vi "samletrev1.vi"() -> ()   [LabVIEW 2019]
uses:
  <vilib>/myRIO/Instrument Drivers/Onboard IO/AI/typedefs/AI Reference.ctl
  <vilib>/myRIO/Common/Instrument Driver Framework/Utilities/typedefs/myRIO Generic Hardware Reference.ctl
  <vilib>/myRIO/Common/Instrument Driver Framework/Utilities/typedefs/Hardware Version Enum.ctl
  <vilib>/myRIO/Common/Instrument Driver Framework/Utilities/typedefs/myRIO v1.0 Reference.ctl
  <vilib>/myRIO/Common/Instrument Driver Framework/Utilities/typedefs/Generic FPGA Reference.ctl
  <vilib>/myRIO/Common/Instrument Driver Framework/myRIO v1.0/AI/typedefs/AI Channels List.ctl
  <vilib>/myRIO/Common/Instrument Driver Framework/myRIO v1.0/AI/typedefs/AI Channels Enum.ctl
  <vilib>/myRIO/Common/Instrument Driver Framework/Utilities/typedefs/Analog Scaling Constants List.ctl
  <vilib>/myRIO/Common/Instrument Driver Framework/Utilities/typedefs/Analog Scaling Constants.ctl
  <vilib>/userdefined/High Color/nirio_resource_hc.ctl
  <vilib>/myRIO/Common/Instrument Driver Framework/myRIO v1.0/Encoder/typedefs/Encoder Signal Mode.ctl
  <vilib>/myRIO/Instrument Drivers/Onboard IO/Encoder/typedefs/Encoder Reference.ctl
  <vilib>/myRIO/Common/Instrument Driver Framework/myRIO v1.0/Encoder/typedefs/Encoder Channels Enum.ctl
  <vilib>/myRIO/Common/Instrument Driver Framework/myRIO v1.0/Encoder/typedefs/Encoder Configuration v1.0.ctl
  <vilib>/myRIO/Instrument Drivers/Onboard IO/PWM/typedefs/PWM Reference.ctl
  <vilib>/myRIO/Common/Instrument Driver Framework/myRIO v1.0/PWM/typedefs/PWM Channels Enum.ctl
  <vilib>/myRIO/Instrument Drivers/Onboard IO/PWM/typedefs/PWM Configuration.ctl
  <vilib>/myRIO/Common/Instrument Driver Framework/Utilities/vis/Is FPGA Ref Available.vi
  <vilib>/myRIO/Common/Instrument Driver Framework/myRIO v1.0/AI/vis/myRIO v1.1 Open AI.vi
  <vilib>/myRIO/Instrument Drivers/Onboard IO/AI/vis/Read.vi
  <vilib>/myRIO/Common/Instrument Driver Framework/myRIO v1.0/Encoder/vis/myRIO v1.1 Open Encoder.vi
  <vilib>/myRIO/Instrument Drivers/Onboard IO/Encoder/vis/Read.vi
  <vilib>/myRIO/Common/Instrument Driver Framework/myRIO v1.0/PWM/vis/myRIO v1.1 Open PWM.vi
  <vilib>/myRIO/Common/Instrument Driver Framework/Utilities/vis/Validate Channels.vi
  <vilib>/myRIO/Common/Instrument Driver Framework/myRIO v1.0/AI/vis/myRIO v1.0 Reserve AI.vi
  <vilib>/myRIO/Common/Instrument Driver Framework/myRIO v1.0/Encoder/vis/myRIO v1.0 Reserve Encoder.vi
  <vilib>/myRIO/Common/Instrument Driver Framework/myRIO v1.0/PWM/vis/myRIO v1.0 Reserve PWM.vi
  <vilib>/myRIO/Common/Instrument Driver Framework/myRIO v1.0/PWM/vis/myRIO v1.0 Close PWM.vi
  <vilib>/myRIO/Common/Instrument Driver Framework/myRIO v1.0/AI/vis/myRIO v1.0 Build MUX Configuration AI.vi
  <vilib>/myRIO/Common/Instrument Driver Framework/myRIO v1.0/Resource Manager/vis/myRIO v1.0 Reserve Channel List.vi
  <vilib>/myRIO/Common/Instrument Driver Framework/myRIO v1.0/Encoder/vis/myRIO v1.0 Build MUX Configuration Encoder.vi
  <vilib>/myRIO/Common/Instrument Driver Framework/myRIO v1.0/PWM/vis/myRIO v1.0 Build MUX Configuration PWM.vi
  <vilib>/myRIO/Common/Instrument Driver Framework/myRIO v1.0/PWM/vis/myRIO v1.0 Unreserve PWM.vi
  <vilib>/myRIO/Common/Instrument Driver Framework/myRIO v1.0/Resource Manager/vis/myRIO v1.0 Reserve Channel.vi
  <vilib>/myRIO/Common/Instrument Driver Framework/myRIO v1.0/Resource Manager/vis/myRIO v1.0 Unreserve Channel.vi
  <vilib>/myRIO/Common/Instrument Driver Framework/myRIO v1.0/Resource Manager/vis/myRIO v1.0 Create Configuration List.vi
  <vilib>/myRIO/Common/Instrument Driver Framework/myRIO v1.0/Resource Manager/vis/myRIO v1.0 Unreserve Channel List.vi
  <vilib>/myRIO/Common/Instrument Driver Framework/myRIO v1.0/Resource Manager/vis/myRIO v1.0 Build Mutex Name.vi
  <vilib>/Utility/VariantDataType/GetNumericInfo.vi
  <vilib>/Utility/error.llb/Error Cluster From Error Code.vi
  <vilib>/myRIO/Common/Instrument Driver Framework/myRIO v1.0/myRIO v1.1 Open.vi
  <vilib>/myRIO/Common/Instrument Driver Framework/Utilities/vis/IO Manager.vi
  <vilib>/myRIO/Common/Instrument Driver Framework/Utilities/vis/Configuration Manager.vi
  <vilib>/myRIO/Common/Instrument Driver Framework/myRIO v1.0/Resource Manager/vis/myRIO v1.0 Configure IO.vi
  <vilib>/myRIO/Common/Instrument Driver Framework/myRIO v1.0/myRIO v1.0 Close.vi
  <vilib>/myRIO/Common/Instrument Driver Framework/myRIO v1.0/PWM/vis/myRIO v1.0 Write PWM.vi
  <vilib>/myRIO/Common/Instrument Driver Framework/myRIO v1.0/PWM/vis/myRIO v1.0 Shutdown PWM.vi
  <vilib>/myRIO/Common/Instrument Driver Framework/myRIO v1.0/Encoder/vis/myRIO v1.0 Configure Encoder.vi
  <vilib>/myRIO/Common/Instrument Driver Framework/myRIO v1.0/Encoder/vis/myRIO v1.0 Read Encoder.vi
  <vilib>/myRIO/Common/Instrument Driver Framework/myRIO v1.0/AI/vis/myRIO v1.0 Get Scaling Constants AI.vi
  <vilib>/myRIO/Common/Instrument Driver Framework/myRIO v1.0/AI/vis/myRIO v1.0 Read AI.vi
  <vilib>/addons/control/pid/pid.llb/PID (DBL).vi
  <vilib>/myRIO/Instrument Drivers/Onboard IO/PWM/vis/myRIO PWM Open.xnode
  <vilib>/myRIO/Express VI/Onboard IO/Encoder/Encoder Express VI.xnode
  <vilib>/myRIO/Instrument Drivers/Onboard IO/Encoder/vis/myRIO Encoder Open.xnode
  <vilib>/myRIO/Common/Instrument Driver Framework/myRIO v1.0/Encoder/typedefs/Encoder Count Direction Enum.ctl
  <vilib>/myRIO/Express VI/Onboard IO/AI/AI Express VI.xnode
  <vilib>/myRIO/Instrument Drivers/Onboard IO/AI/vis/myRIO AI Open.xnode
  <vilib>/myRIO/Instrument Drivers/Onboard IO/PWM/PWM.lvlib
  <vilib>/myRIO/Instrument Drivers/Onboard IO/Encoder/Encoder.lvlib
  <vilib>/ptbypt/NI_PtbyPt.lvlib
  <vilib>/myRIO/Instrument Drivers/Onboard IO/AI/AI.lvlib
  <vilib>/addons/control/pid/NI_PID_pid.lvlib
panel:
  in  "y":dbl
  out "output":dbl format="%.2f"
  in  "PWM-treshold":dbl format="%#_13g"
  out "PWM-sig":dbl format="%.2f"
  in  "1-output range":cluster{"output high":dbl, "output low":dbl}={"output high"=100.0, "output low"=-100.0} {"output low" format="%.2f"; "output high" format="%.2f"}
  in  "PID-1 gains":T1={"proportional gain (Kc)"=1.0, "integral time (Ti, min)"=0.01, "derivative time (Td, min)"=0.0} {"derivative time (Td, min)" format="%.3f"; "integral time (Ti, min)" format="%.3f"; "proportional gain (Kc)" format="%.3f"}
  out "x(F.R) test":dbl
  out "x(F.L) test":dbl
  in  "stop":bool
  out "Front  Left(F.L)":T2(graph)
  out "Sensor 1":dbl=0.0038137989155123176 format="%0.5f"
  in  "ZERO ALL SENSORS":bool
  in  "STOP SYSTEM":bool
  out "Sensor 2":dbl=0.0038137989155123176 format="%0.5f"
  out "Front  Right(F.L)":T2(graph)
  out "Sensor 3":dbl=0.0038137989155123176 format="%0.5f"
  out "Back Left(F.L)":T2(graph)
  out "Sensor 4":dbl=0.0038137989155123176 format="%0.5f"
  out "Back Right(F.L)":T2(graph)
  out "Sensor 5":dbl=0.0038137989155123176 format="%0.5f"
  out "Front Left(F.R)":T2(graph)
  out "Sensor 6":dbl=0.0038137989155123176 format="%0.5f"
  out "Front Right(F.R)":T2(graph)
  out "Sensor 7":dbl=0.0038137989155123176 format="%0.5f"
  out "Back Left(F.R)":T2(graph)
  out "Sensor 8":dbl=0.0038137989155123176 format="%0.5f"
  out "Back Right(F.R)":T2(graph)
  out "Sensor 9":dbl=0.0038137989155123176 format="%0.5f"
  out "Axial(L)":T2(graph)
  out "Sensor 10":dbl=0.0038137989155123176 format="%0.5f"
  out "Axial(R)":T2(graph)
  in  "Cal(F.L)":dbl[](array[numeric])
  out "Kg(L)":dbl[](array[numeric])
  out "Sum(L)":dbl
  in  "Cal(F.R)":dbl[](array[numeric])
  out "Kg (R)":dbl[](array[numeric])
  out "Sum(R)":dbl
  out "x(F.R)":dbl
  out "y(F.R)":dbl
  out "sum(F.R)":dbl
  out "Sum (F.L)":dbl
  out "y(F.L)":dbl
  out "x(F.L)":dbl
  out "Cop Left":cluster{dbl[], dbl[]}(graph)
  out "Cop Right":cluster{dbl[], dbl[]}(graph)
  in  "x Right":dbl[](array[numeric])
  in  "kal Right":dbl=1.0
  in  "x Left":dbl[](array[numeric])
  in  "kal left":dbl=1.0
  in  "Stop":bool
  in  "Reset Counter":bool
  out "Counter Value Right":i32
  out "Pulstime Right":u32
  out "km/h Right belt":dbl(knob) scale=0.0..15.0
  out "km/h 2":dbl format="%#_2g"
  out "Counter Value left":i32
  out "Pulstime left":u32
  out "km/h left belt":dbl(knob) scale=0.0..15.0
  out "km/h":dbl format="%#_2g"
  in  "STOP RIGHT MOTOR":bool
  in  "RIGHT MOTOR DUTY CYCLE":dbl(slide)=50.00000000000001 scale=0.0..100.0
  in  "STOP LEFT MOTOR":bool
  in  "LEFT MOTOR DUTY CYCLE":dbl(slide)=50.00000000000001 scale=0.0..100.0
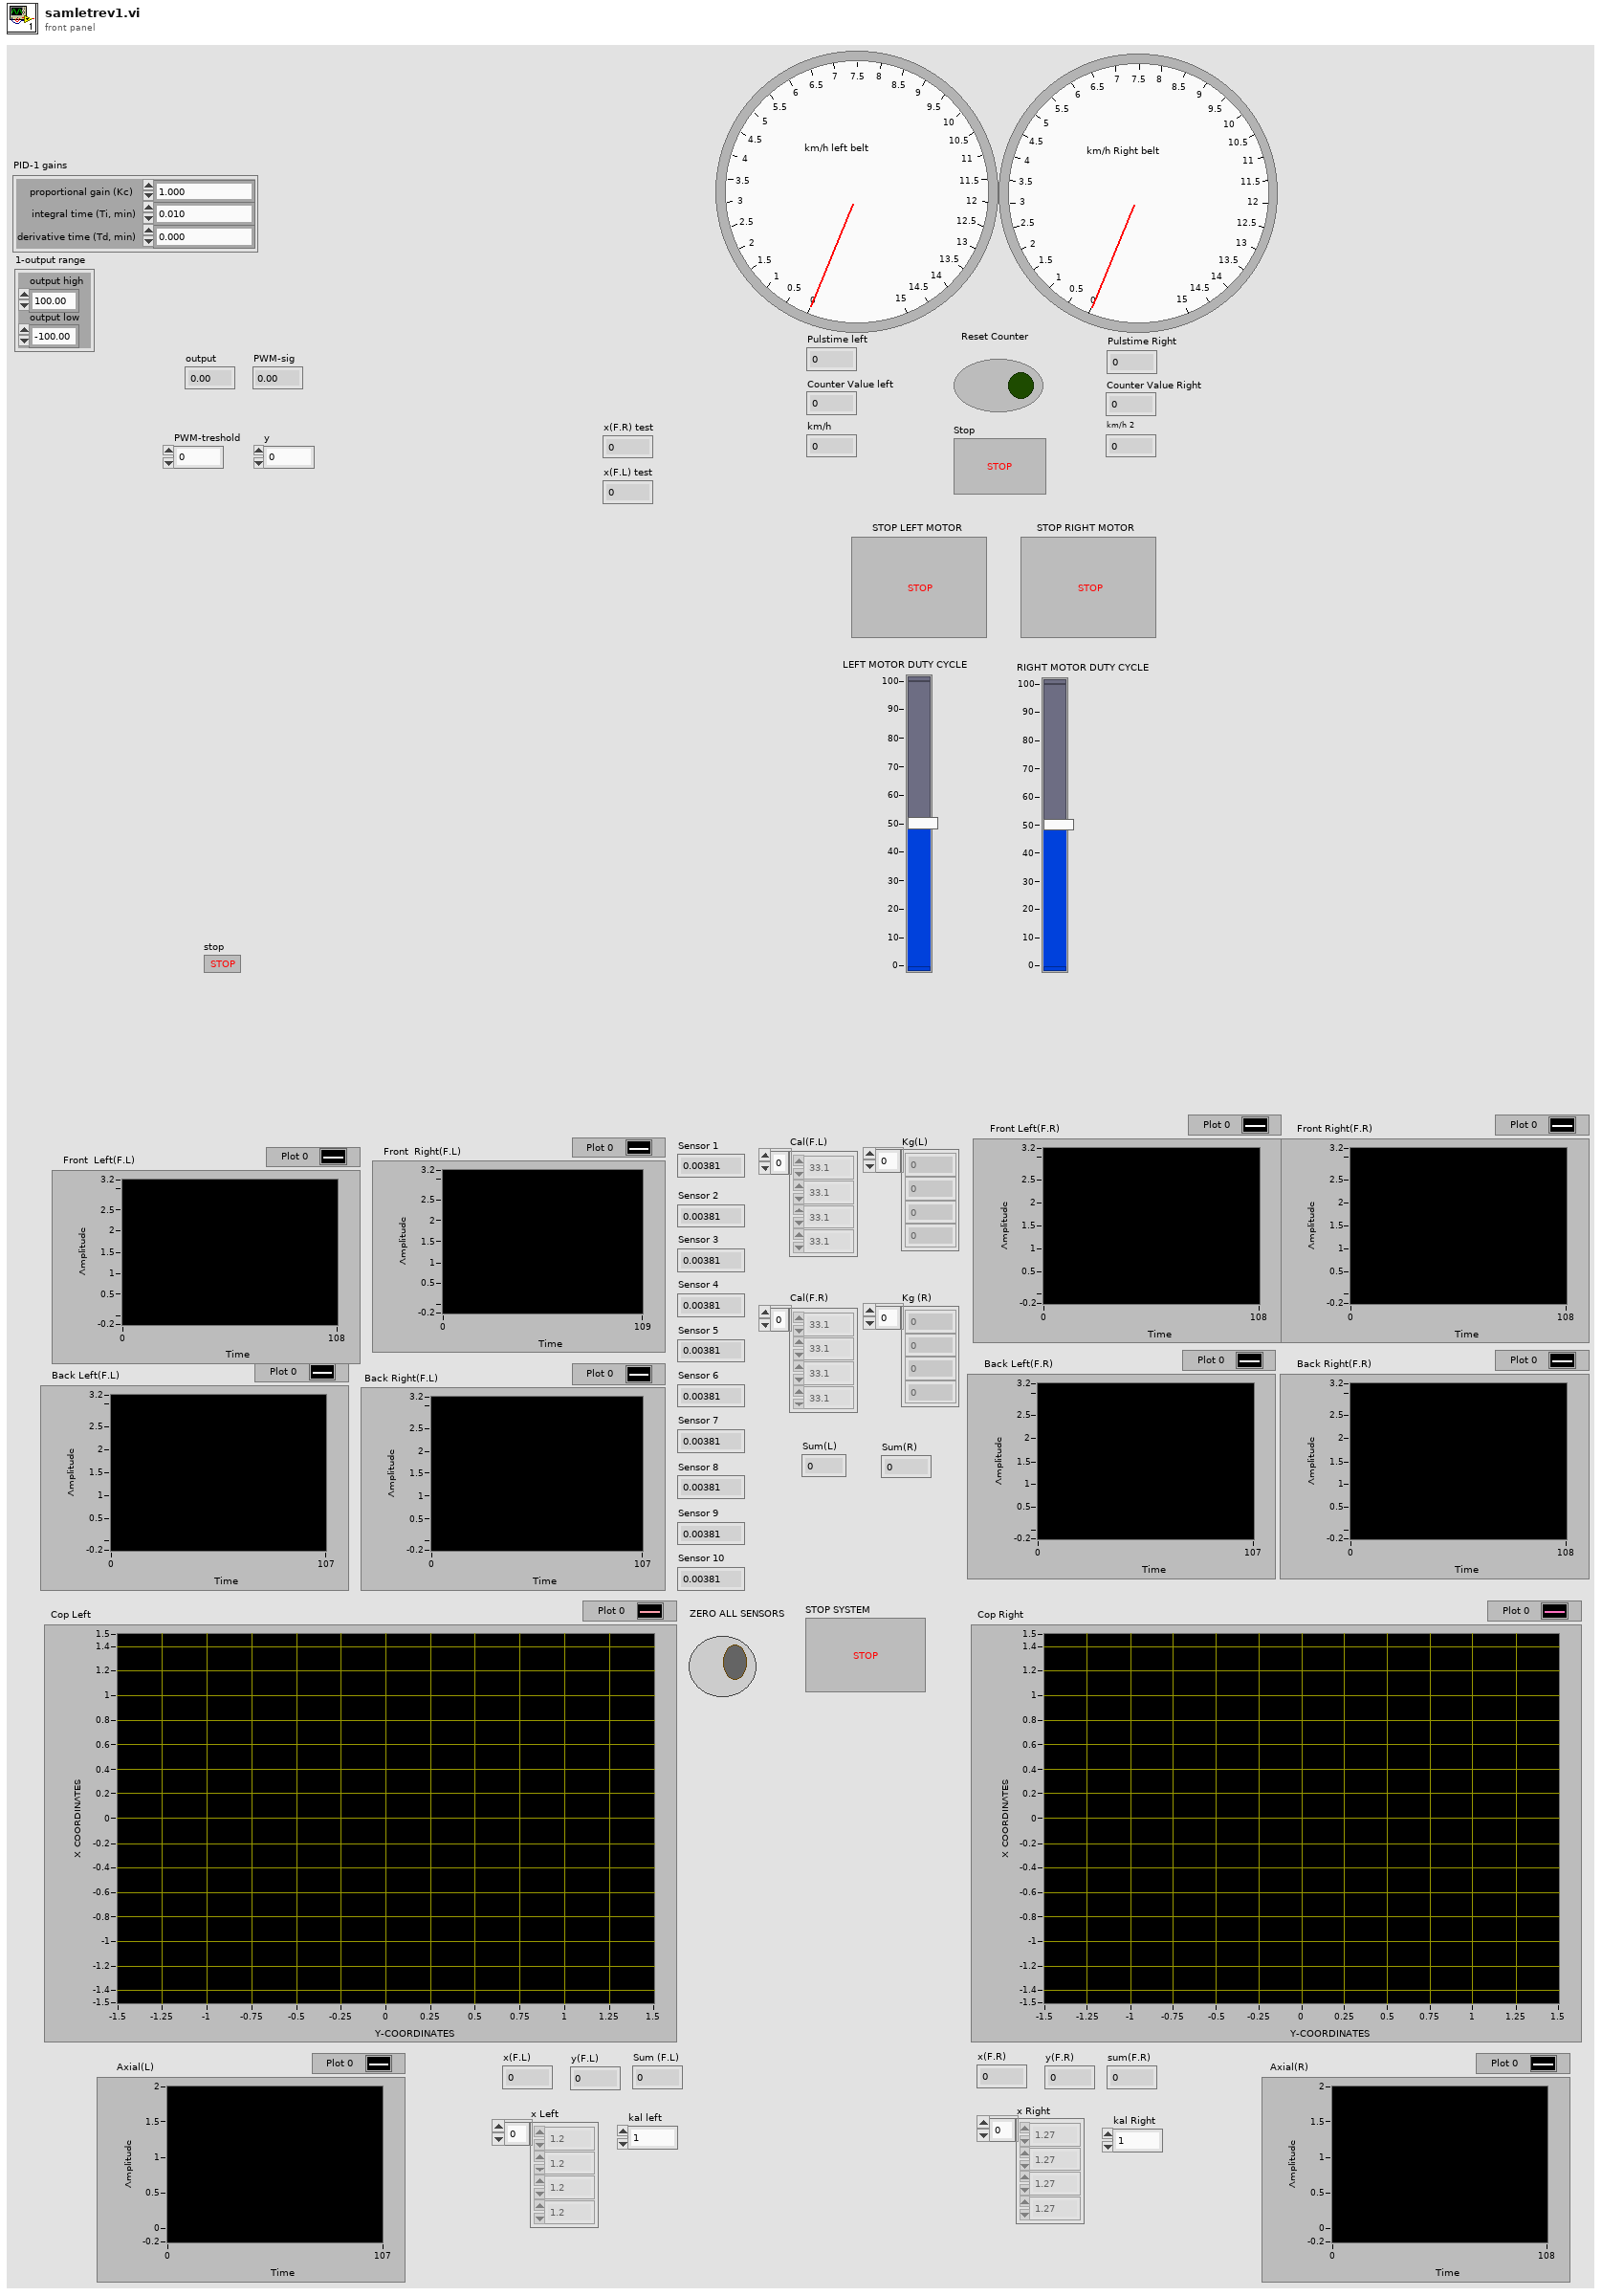
[diagram p1: front panel]
types:
  T1 = cluster{"proportional gain (Kc)":dbl, "integral time (Ti, min)":dbl, "derivative time (Td, min)":dbl}
  T2 = cluster{"Filtered x":dbl, "Sensor 1 (A/AI0 (Pin 3))":dbl}
  T3 = typedef "PWM.lvlib/PWM Reference.ctl" = cluster{"myRIO Reference":T4, "PWM Channels Enum":T8, "PWM Configuration":T9}
  T4 = typedef "myRIO Generic Hardware Reference.ctl" = cluster{"myRIO Model":T5, "myRIO Hardware Reference":T6}
  T5 = typedef "Hardware Version Enum.ctl" = enum16{"Unknown", "myRIO-1900", "myRIO-1950", "roboRIO", "NI ELVIS RIO CM", "ELVIS III"}
  T6 = typedef "myRIO v1.0 Reference.ctl" = cluster{"Generic FPGA Reference":T7, "Allow multiple opens":bool}
  T7 = typedef "Generic FPGA Reference.ctl" = refnum<k20>
  T8 = typedef "PWM Channels Enum.ctl" = enum16{"Not Connected", "C/PWM0", "C/PWM1", "A/PWM0", "A/PWM1", "A/PWM2", "A/PWM3", "A/PWM4", "A/PWM5", "A/PWM6", "A/PWM7", "A/PWM8", "A/PWM9", "A/PWM10", "A/PWM11", "A/PWM12", "A/PWM13", "A/PWM14", "A/PWM15", "A/PWM16", "A/PWM17", "A/PWM18", "A/PWM19", "B/PWM0", "B/PWM1", "B/PWM2", "B/PWM3", "B/PWM4", "B/PWM5", "B/PWM6", "B/PWM7", "B/PWM8", "B/PWM9", "B/PWM10", "B/PWM11", "B/PWM12", "B/PWM13", "B/PWM14", "B/PWM15", "B/PWM16", "B/PWM17", "B/PWM18", "B/PWM19", "PWM/PWM0", "PWM/PWM1", "PWM/PWM2", "PWM/PWM3", "PWM/PWM4", "PWM/PWM5", "PWM/PWM6", "PWM/PWM7", "PWM/PWM8", "PWM/PWM9"}
  T9 = typedef "PWM.lvlib/PWM Configuration.ctl" = cluster{"Frequency":dbl, "Duty Cycle":dbl}
  T10 = typedef "Encoder.lvlib/Encoder Reference.ctl" = cluster{"myRIO Reference":T4, "Encoder Channels Enum":T11}
  T11 = typedef "Encoder Channels Enum.ctl" = enum16{"Not Connected", "C/ENC0", "C/ENC1", "A/ENC", "A/ENC0", "A/ENC1", "A/ENC2", "A/ENC3", "A/ENC4", "A/ENC5", "A/ENC6", "A/ENC7", "A/ENC8", "A/ENC9", "B/ENC", "B/ENC0", "B/ENC1", "B/ENC2", "B/ENC3", "B/ENC4", "B/ENC5", "B/ENC6", "B/ENC7", "B/ENC8", "B/ENC9", "DIO/ENC0", "DIO/ENC1", "DIO/ENC2", "DIO/ENC3", "DIO/ENC4"}
  T12 = typedef "Encoder Signal Mode.ctl" = enum16{"Quadrature phase signal", "Step and direction signal"}
  T13 = typedef "nirio_resource_hc.ctl" = tag
  T14 = typedef "AI.lvlib/AI Reference.ctl" = cluster{"myRIO Reference":T4, "AI Channels List":T15, "AI Scaling Constants List":T17}
  T15 = typedef "AI Channels List.ctl" = T16[]
  T16 = typedef "AI Channels Enum.ctl" = enum16{"Not Connected", "AudioIn/Left", "AudioIn/Right", "C/AI0", "C/AI1", "A/AI0", "A/AI1", "A/AI2", "A/AI3", "A/AI4", "A/AI5", "A/AI6", "A/AI7", "B/AI0", "B/AI1", "B/AI2", "B/AI3", "B/AI4", "B/AI5", "B/AI6", "B/AI7", "AI/AI0", "AI/AI1", "AI/AI2", "AI/AI3", "A/AI0 (DIFF)", "A/AI1 (DIFF)", "A/AI2 (DIFF)", "A/AI3 (DIFF)", "B/AI0 (DIFF)", "B/AI1 (DIFF)", "B/AI2 (DIFF)", "B/AI3 (DIFF)"}
  T17 = typedef "Analog Scaling Constants List.ctl" = T18[]
  T18 = typedef "Analog Scaling Constants.ctl" = cluster{"LSB Weight (Volts)":dbl, "Offset (Volts)":dbl, "Signed?":bool}
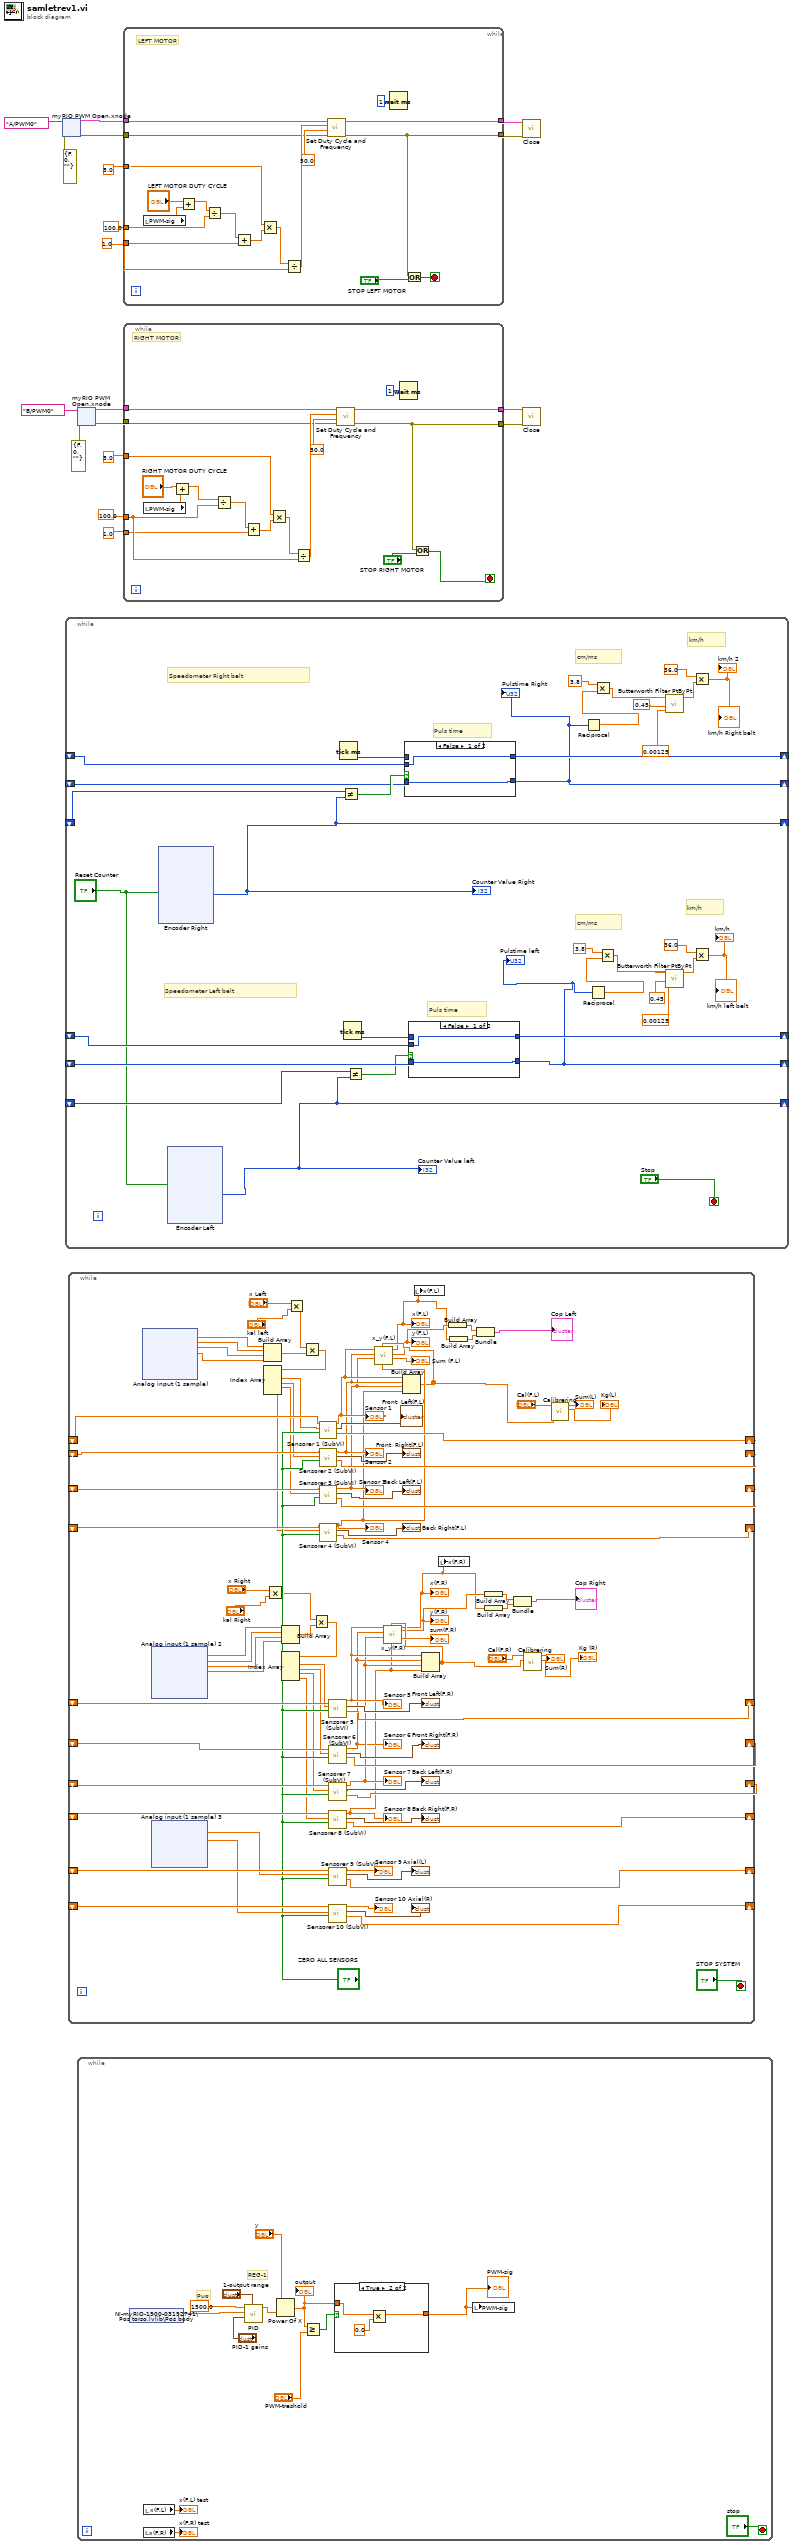
[diagram p0: block diagram]
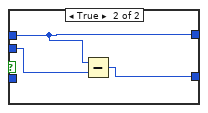
[diagram p3: hidden frame]
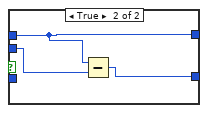
[diagram p4: hidden frame]
diagram:
  n1 = xnode "myRIO PWM Open.xnode"("error in (no error)"=errorcluster {"status"=FALSE, "code"=0, "source"=""}, "Channel Name"=tag "A/PWM0") -> ("error out"=w15:errorcluster, "PWM Ref Out"=w2:T3)  [unwired: 1 in]
  n2 = while {
    shift-right: [w20] -> _
    shift-left: _ -> [w51]
    shift-right: [w49] -> _
    shift-left: _ -> [w47]
    shift-right: [w22] -> _
    shift-left: _ -> [w46]
    shift-right: [w21] -> _
    shift-left: _ -> [w33]
    shift-right: [w25] -> _
    shift-left: _ -> [w36]
    shift-right: [w24] -> _
    shift-left: _ -> [w37]
    stop <- "Stop" stop-if-true
    # "Puls time"
    # "Puls time"
    # "km/h"
    # "cm/ms"
    # "km/h"
    # "cm/ms"
    # "Speedometer Left belt"
    # "Speedometer Right belt"
    n3 = xnode "Encoder Right"("Reset Counter"="Reset Counter") -> ("Counter Value"=w20:i32)  [unwired: 1 in, 3 out]
    "Counter Value Right" <- w20
    n4 = xnode "Encoder Left"("Reset Counter"="Reset Counter") -> ("Counter Value"=w21:i32)  [unwired: 1 in, 3 out]
    "Counter Value left" <- w21
    n5 = Tick Count (ms)() -> (millisecond timer value=w48:u32)
    n6 = Not Equal?(x=w51, y=w20) -> (x != y?=w50:bool)
    n7 = Tick Count (ms)() -> (millisecond timer value=w35:u32)
    n8 = Not Equal?(x=w33, y=w21) -> (x != y?=w34:bool)
    n9 = case shown="False" w50 {
      tunnel: [w105 w108] -> w49
      tunnel: w48 -> [_ w108]
      tunnel: w47 -> [w105 w107]
      tunnel: [w104 w106] -> w22
      tunnel: w46 -> [w104 _]
      frame False {
      }
      frame True {
        n10 = Subtract(x=w108, y=w107) -> (x-y=w106:u32)
      }
    }
    "Pulstime Right" <- w22
    n11 = case shown="False" w34 {
      tunnel: [w54 w57] -> w25
      tunnel: w35 -> [_ w57]
      tunnel: w36 -> [w54 w56]
      tunnel: [w53 w55] -> w24
      tunnel: w37 -> [w53 _]
      frame False {
      }
      frame True {
        n12 = Subtract(x=w57, y=w56) -> (x-y=w55:u32)
      }
    }
    "Pulstime left" <- w24
    n13 = Reciprocal(x=w22) -> (1/x=w45:dbl)
    n14 = Reciprocal(x=w24) -> (1/x=w26:dbl)
    n15 = Multiply(x=3.8, y=w45) -> (x*y=w44:dbl)
    n16 = Multiply(x=3.8, y=w26) -> (x*y=w19:dbl)
    n17 = call <vilib>:"Butterworth Filter PtByPt.vi"("low cutoff freq: fl"=0.00125, "high cutoff freq: fh"=0.45, "x"=w19) -> ("Filtered x"=w30:dbl)  [unwired: 6 in, 1 out]
    n18 = call <vilib>:"Butterworth Filter PtByPt.vi"("low cutoff freq: fl"=0.00125, "high cutoff freq: fh"=0.45, "x"=w44) -> ("Filtered x"=w40:dbl)  [unwired: 6 in, 1 out]
    n19 = Multiply(x=36.0, y=w40) -> (x*y=→"km/h Right belt" →"km/h 2":dbl)
    n20 = Multiply(x=36.0, y=w30) -> (x*y=→"km/h left belt" →"km/h":dbl)
  }
  n21 = while {
    shift-right: [w207] -> _
    shift-left: _ -> [w237]
    shift-right: [w205] -> _
    shift-left: _ -> [w236]
    shift-right: [w203] -> _
    shift-left: _ -> [w234]
    shift-right: [w206] -> _
    shift-left: _ -> [w232]
    shift-right: [w211] -> _
    shift-left: _ -> [w230]
    shift-right: [w210] -> _
    shift-left: _ -> [w228]
    shift-right: [w209] -> _
    shift-left: _ -> [w226]
    shift-right: [w208] -> _
    shift-left: _ -> [w224]
    shift-right: [w218] -> _
    shift-left: _ -> [w222]
    shift-right: [w212] -> _
    shift-left: _ -> [w217]
    stop <- "STOP SYSTEM" stop-if-true
    n22 = xnode "Analog input (1 sample)"() -> ("Sensor 1 (A/AI0 (Pin 3))"=w173:dbl, "Sensor 2 (A/AI1 (Pin 5))"=w172:dbl, "Sensor 3 (A/AI2 (Pin 7))"=w171:dbl, "Sensor 4 (A/AI3 (Pin 9))"=w170:dbl)  [unwired: 1 in, 1 out]
    n23 = xnode "Analog input (1 sample) 2"() -> ("Sensor 5 (B/AI0 (Pin 3))"=w182:dbl, "Sensor 6 (B/AI1 (Pin 5))"=w180:dbl, "Sensor 7 (B/AI2 (Pin 7))"=w159:dbl, "Sensor 8 (B/AI3 (Pin 9))"=w169:dbl)  [unwired: 1 in, 1 out]
    n24 = xnode "Analog input (1 sample) 3"() -> ("Sensor 9 (C/AI0 (AI0))"=w221:dbl, "Sensor 10 (C/AI1 (AI1))"=w216:dbl)  [unwired: 1 in, 1 out]
    n25 = Build Array(w173, w172, w171, w170) -> (w162:dbl[])
    n26 = Multiply(x="x Right", y="kal Right") -> (x*y=w176:dbl[])
    n27 = Build Array(w182, w180, w159, w169) -> (w185:dbl[])
    n28 = Multiply(x="x Left", y="kal left") -> (x*y=w161:dbl[])
    n29 = Multiply(x=w161, y=w162) -> (x*y=w160:dbl[])
    n30 = Index Array(array=w160) -> (element #1=w166:dbl, element #2=w165:dbl, element #3=w164:dbl, element #4=w163:dbl)  [unwired: 4 in]
    n31 = Multiply(x=w176, y=w185) -> (x*y=w183:dbl[])
    n32 = Index Array(array=w183) -> (element #1=w181:dbl, element #2=w179:dbl, element #3=w178:dbl, element #4=w177:dbl)  [unwired: 4 in]
    n33 = call "Sensorer 1 (SubVI).vi"("ZERO ALL SENSORS"="ZERO ALL SENSORS", "Sensor 3 (A/AI2(Pin7))"=w166, "Filtered x in"=w237) -> ("Filtered x out"=w207:dbl, "F.L Rear Leftt"=→"Front  Left(F.L)":T2, "Sensor 1"=w197:dbl)  [unwired: 6 in]
    "Sensor 1" <- w197
    n34 = call "Sensorer 2 (SubVI).vi"("ZERO ALL SENSORS"="ZERO ALL SENSORS", "Sensor 3 (A/AI2(Pin7))"=w165, "Filtered x in"=w236) -> ("Filtered x out"=w205:dbl, "F.L Rear Leftt"=→"Front  Right(F.L)":T2, "Sensor 1"=w196:dbl)  [unwired: 6 in]
    "Sensor 2" <- w196
    n35 = call "Sensorer 3 (SubVI).vi"("ZERO ALL SENSORS"="ZERO ALL SENSORS", "Sensor 3 (A/AI2(Pin7))"=w164, "Filtered x in"=w234) -> ("Filtered x out"=w203:dbl, "F.L Rear Leftt"=→"Back Left(F.L)":T2, "Sensor 1"=w195:dbl)  [unwired: 6 in]
    "Sensor 3" <- w195
    n36 = call "Sensorer 4 (SubVI).vi"("ZERO ALL SENSORS"="ZERO ALL SENSORS", "Sensor 3 (A/AI2(Pin7))"=w163, "Filtered x in"=w232) -> ("Filtered x out"=w206:dbl, "F.L Rear Leftt"=→"Back Right(F.L)":T2, "Sensor 1"=w194:dbl)  [unwired: 6 in]
    "Sensor 4" <- w194
    n37 = call "Sensorer 5 (SubVI).vi"("ZERO ALL SENSORS"="ZERO ALL SENSORS", "Sensor 3 (A/AI2(Pin7))"=w181, "Filtered x in"=w230) -> ("Filtered x out"=w211:dbl, "F.L Rear Leftt"=→"Front Left(F.R)":T2, "Sensor 1"=w201:dbl)  [unwired: 6 in]
    "Sensor 5" <- w201
    n38 = call "Sensorer 6 (SubVI).vi"("ZERO ALL SENSORS"="ZERO ALL SENSORS", "Sensor 3 (A/AI2(Pin7))"=w179, "Filtered x in"=w228) -> ("Filtered x out"=w210:dbl, "F.L Rear Leftt"=→"Front Right(F.R)":T2, "Sensor 1"=w199:dbl)  [unwired: 6 in]
    "Sensor 6" <- w199
    n39 = call "Sensorer 7 (SubVI).vi"("ZERO ALL SENSORS"="ZERO ALL SENSORS", "Sensor 3 (A/AI2(Pin7))"=w178, "Filtered x in"=w226) -> ("Filtered x out"=w209:dbl, "F.L Rear Leftt"=→"Back Left(F.R)":T2, "Sensor 1"=w200:dbl)  [unwired: 6 in]
    "Sensor 7" <- w200
    n40 = call "Sensorer 8 (SubVI).vi"("ZERO ALL SENSORS"="ZERO ALL SENSORS", "Sensor 3 (A/AI2(Pin7))"=w177, "Filtered x in"=w224) -> ("Filtered x out"=w208:dbl, "F.L Rear Leftt"=→"Back Right(F.R)":T2, "Sensor 1"=w198:dbl)  [unwired: 6 in]
    "Sensor 8" <- w198
    n41 = call "Sensorer 9 (SubVI).vi"("ZERO ALL SENSORS"="ZERO ALL SENSORS", "Sensor 3 (A/AI2(Pin7))"=w221, "Filtered x in"=w222) -> ("Filtered x out"=w218:dbl, "F.L Rear Leftt"=→"Axial(L)":T2, "Sensor 1"=→"Sensor 9":dbl)  [unwired: 6 in]
    n42 = call "Sensorer 10 (SubVI).vi"("ZERO ALL SENSORS"="ZERO ALL SENSORS", "Sensor 3 (A/AI2(Pin7))"=w216, "Filtered x in"=w217) -> ("Filtered x out"=w212:dbl, "F.L Rear Leftt"=→"Axial(R)":T2, "Sensor 1"=→"Sensor 10":dbl)  [unwired: 6 in]
    n43 = Build Array(w197, w196, w195, w194) -> (w186:dbl[])
    n44 = call "x_y(F.L).vi"("Sensor 4"=w194, "Array"=w186, "Sensor 3"=w195, "Sensor 2"=w196, "Sensor 1"=w197) -> ("Sum (F.L)"=→"Sum (F.L)":dbl, "y(F.L)"=w158:dbl, "x(F.L)"=w155:dbl)  [unwired: 4 in]
    "y(F.L)" <- w158
    "x(F.L)" <- w155
    n45 = local write "x(F.L)"(w155) -> ()
    n46 = Build Array(w201, w199, w200, w198) -> (w192:dbl[])
    n47 = call "x_y(F.R).vi"("Sensor 8"=w198, "Array"=w192, "Sensor 7"=w200, "Sensor 6"=w199, "Sensor 5"=w201) -> ("Sum(F.R)"=→"sum(F.R)":dbl, "y(F.R)"=w174:dbl, "x(F.R)"=w156:dbl)  [unwired: 4 in]
    "x(F.R)" <- w156
    "y(F.R)" <- w174
    n48 = local write "x(F.R)"(w156) -> ()
    n49 = Build Array(w158) -> (w191:dbl[])
    n50 = Build Array(w155) -> (w188:dbl[])
    n51 = Bundle(w191, w188) -> (→"Cop Left":cluster{dbl[], dbl[]})  [unwired: 1 in]
    n52 = Build Array(w174) -> (w190:dbl[])
    n53 = Build Array(w156) -> (w189:dbl[])
    n54 = Bundle(w190, w189) -> (→"Cop Right":cluster{dbl[], dbl[]})  [unwired: 1 in]
    n55 = call "Calibrering.vi"("Array"=w192, "Cal(F.L)"="Cal(F.R)") -> ("Kg"=→"Kg (R)":dbl[], "sum"=→"Sum(R)":dbl)  [unwired: 8 in]
    n56 = call "Calibrering.vi"("Array"=w186, "Cal(F.L)"="Cal(F.L)") -> ("Kg"=→"Kg(L)":dbl[], "sum"=→"Sum(L)":dbl)  [unwired: 8 in]
  }
  n57 = xnode "myRIO PWM Open.xnode"("error in (no error)"=errorcluster {"status"=FALSE, "code"=0, "source"=""}, "Channel Name"=tag "B/PWM0") -> ("error out"=w1:errorcluster, "PWM Ref Out"=w4:T3)  [unwired: 1 in]
  n58 = while {
    stop <- "stop" stop-if-true
    # "REG-1"
    # "Puø"
    n59 = shared-variable "NI-myRIO-1900-03192741\\Pos torso.lvlib\\Pos body"() -> (w371:dbl)  [unwired: 1 in, 1 out]
    n60 = local read "x(F.R)"() -> (→"x(F.R) test":dbl)
    n61 = local read "x(F.L)"() -> (→"x(F.L) test":dbl)
    n62 = call-poly <vilib>:"PID.vi"("output range"="1-output range", "PID gains"="PID-1 gains", "process variable"=w371, "setpoint"=1500.0 ("x")) -> ("output"=w365:dbl)  [unwired: 6 in, 1 out]
    n63 = Power Of X(1:w365, 2:"y") -> (0:w364:dbl)
    "output" <- w364
    n64 = Greater Or Equal?(x=w364, y="PWM-treshold") -> (x >= y?=w368:bool)
    n65 = case shown="True" w368 {
      tunnel: w364 -> [w376 w379]
      tunnel: [w376 w378] -> w366
      frame False {
      }
      frame True {
        n66 = Multiply(x=w379, y=0.0) -> (x*y=w378:dbl)
      }
    }
    "PWM-sig" <- w366
    n67 = local write "PWM-sig"(w366) -> ()
  }
  n68 = while {
    tunnel: w2 -> [w391]
    tunnel: [w390] -> w14
    tunnel: [w383] -> w3
    tunnel: w15 -> [w389]
    tunnel: 5.0 ("Numeric 2") -> [w388]
    tunnel: 100.0 ("Numeric") -> [w387]
    tunnel: 1.0 ("Numeric 3") -> [w386]
    stop <- w384 stop-if-true
    # "LEFT MOTOR"
    n69 = local read "PWM-sig"() -> (w380:dbl)
    n70 = Add(x="LEFT MOTOR DUTY CYCLE", y=w380) -> (x+y=w381:dbl)
    n71 = Divide(x=w381, y=w387) -> (x/y=w392:dbl)
    n72 = Add(x=w392, y=w386) -> (x+y=w393:dbl)
    n73 = Multiply(x=w388, y=w393) -> (x*y=w394:dbl)
    n74 = Divide(x=w394, y=w387) -> (x/y=w396:dbl)
    n75 = call <vilib>:"Set Duty Cycle and Frequency.vi"("error in (no error)"=w389, "Frequency [Hz]"=50.0, "Duty Cycle"=w396, "PWM Ref In"=w391) -> ("error out"=w383:errorcluster, "PWM Ref Out"=w390:T3)  [unwired: 5 in]
    n76 = Wait (ms)(milliseconds to wait=u32 1) -> ()  [unwired: 1 out]
    n77 = Or(x=w383, y="STOP LEFT MOTOR") -> (x .or. y?=w384:bool)
  }
  n78 = while {
    tunnel: w4 -> [w409]
    tunnel: [w408] -> w9
    tunnel: [w401] -> w8
    tunnel: w1 -> [w407]
    tunnel: 5.0 ("Numeric 2") -> [w406]
    tunnel: 100.0 ("Numeric") -> [w405]
    tunnel: 1.0 ("Numeric 3") -> [w404]
    stop <- w402 stop-if-true
    # "RIGHT MOTOR"
    n79 = local read "PWM-sig"() -> (w398:dbl)
    n80 = Add(x="RIGHT MOTOR DUTY CYCLE", y=w398) -> (x+y=w399:dbl)
    n81 = Divide(x=w399, y=w405) -> (x/y=w410:dbl)
    n82 = Add(x=w410, y=w404) -> (x+y=w411:dbl)
    n83 = Multiply(x=w406, y=w411) -> (x*y=w412:dbl)
    n84 = Divide(x=w412, y=w405) -> (x/y=w414:dbl)
    n85 = call <vilib>:"Set Duty Cycle and Frequency.vi"("error in (no error)"=w407, "Frequency [Hz]"=50.0, "Duty Cycle"=w414, "PWM Ref In"=w409) -> ("error out"=w401:errorcluster, "PWM Ref Out"=w408:T3)  [unwired: 5 in]
    n86 = Wait (ms)(milliseconds to wait=u32 1) -> ()  [unwired: 1 out]
    n87 = Or(x=w401, y="STOP RIGHT MOTOR") -> (x .or. y?=w402:bool)
  }
  n88 = call <vilib>:"Close.vi"("error in (no error)"=w3, "PWM Ref In"=w14) -> ()  [unwired: 9 in, 1 out]
  n89 = call <vilib>:"Close.vi"("error in (no error)"=w8, "PWM Ref In"=w9) -> ()  [unwired: 9 in, 1 out]
